vi "Get Test Statuses.vi"(11 "Result Model in":refnum<class "Result Model.lvclass">) -> (3 "Test Statuses":map{string, T1}(c390))   [LabVIEW 2020, in "Result Model.lvclass"]
uses:
  Result Model.lvclass
  Result Model.lvclass/Result Model.ctl
  Result/Status.ctl
  Result/Result.lvlib
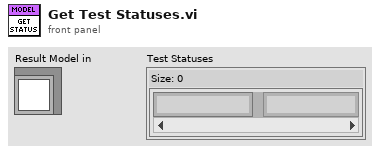
[diagram p1: front panel]
types:
  T1 = typedef "Result.lvlib/Status.ctl" = enum16{"", "Passed", "Failed", "Error", "Skipped", "Setup Error", "Broken", "Teardown Error"}
  T2 = typedef "Result Model.lvclass/Model State.ctl" = cluster{"Run Queue":set{string}, "Test Statuses":map{string, T1}, "Execution Time":map{string, dbl}, "Assertions":map{string, cluster{"Result Type":T3, "Status":T1, "Message":string, "Description":string}[]}}
  T3 = typedef "Result.lvlib/Type.ctl" = enum16{"Method", "Case", "Suite", "Pass", "Fail", "Skip", "Pass if", "Fail if", "Pass if Error", "Fail if Error", "Pass if Equal", "Fail if Equal"}
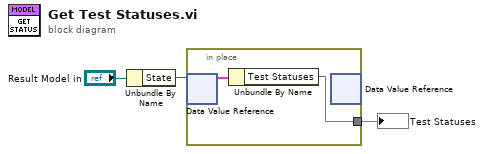
[diagram p0: block diagram]
diagram:
  n1 = Unbundle By Name("Result Model in") -> ("State"=w2:refnum<data-value>)
  n2 = in-place {
    in-place-border: [w4] -> w3
    n3 = in-place-dvr #1(w2) -> (w5:T2)  [unwired: 1 out]
    n4 = Unbundle By Name(w5) -> ("Test Statuses"=w4:map{string, T1})
    n5 = in-place-dvr #1() -> ()  [unwired: 1 in, 2 out]
  }
  "Test Statuses" <- w3
